vi "main.vi"() -> ()   [LabVIEW 2020]
panel:
  in  "Cluster":cluster{}
  in  "5170Rs":void[](array[numeric])
  in  "5764s":void[](array[numeric])
  in  "5172s":void[](array[numeric])
  in  "System":cluster{"Chassi 0":cluster{}}
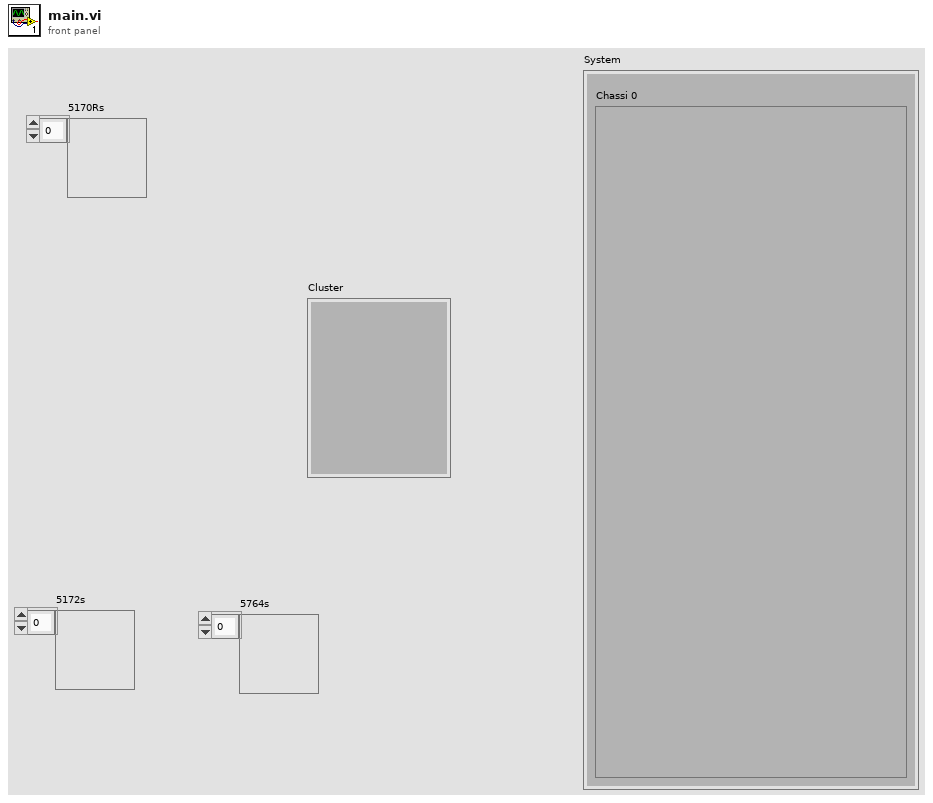
[diagram p1: front panel]
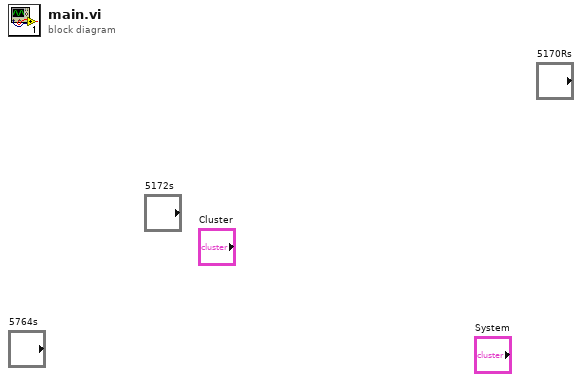
[diagram p0: block diagram]
diagram:
